vi "SMU_Meas and Calculate Resitance.vi"(7 "Current  Level":dbl=0.01, 8 "error in (no error)":errorcluster, 9 "Published Data Id":string, 10 "Pins":string[](array[string]), 11 "Semiconductor Module Context":T1) -> (0 "error Out":errorcluster, 2 "R Array":dbl[](array[numeric]), 3 "Semiconductor Module Context Out":T1)   [LabVIEW 2013]
uses:
  <vilib>/NI_TestStand_SemiconductorModule/NI_TestStand_Semiconductor_Module.lvlibp/PinMap/General/SemiconductorModuleContext.ctl
  <vilib>/NI_TestStand_SemiconductorModule/NI_TestStand_Semiconductor_Module.lvlibp/PinMap/DC Power/PinsToNIDCPowerSessions.vi
  <vilib>/NI_TestStand_SemiconductorModule/NI_TestStand_Semiconductor_Module.lvlibp/PinMap/General/Publish/PublishDataDoubleFunctionalTest.vi
  <vilib>/NI_TestStand_SemiconductorModule/NI_TestStand_Semiconductor_Module.lvlibp
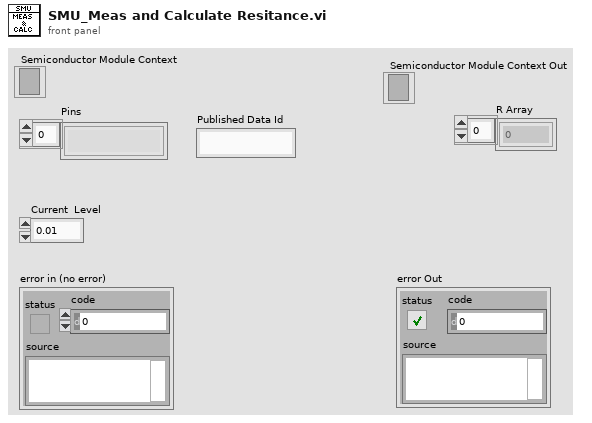
[diagram p1: front panel]
types:
  T1 = typedef "NI_TestStand_Semiconductor_Module.lvlibp/SemiconductorModuleContext.ctl" = refnum<k7>
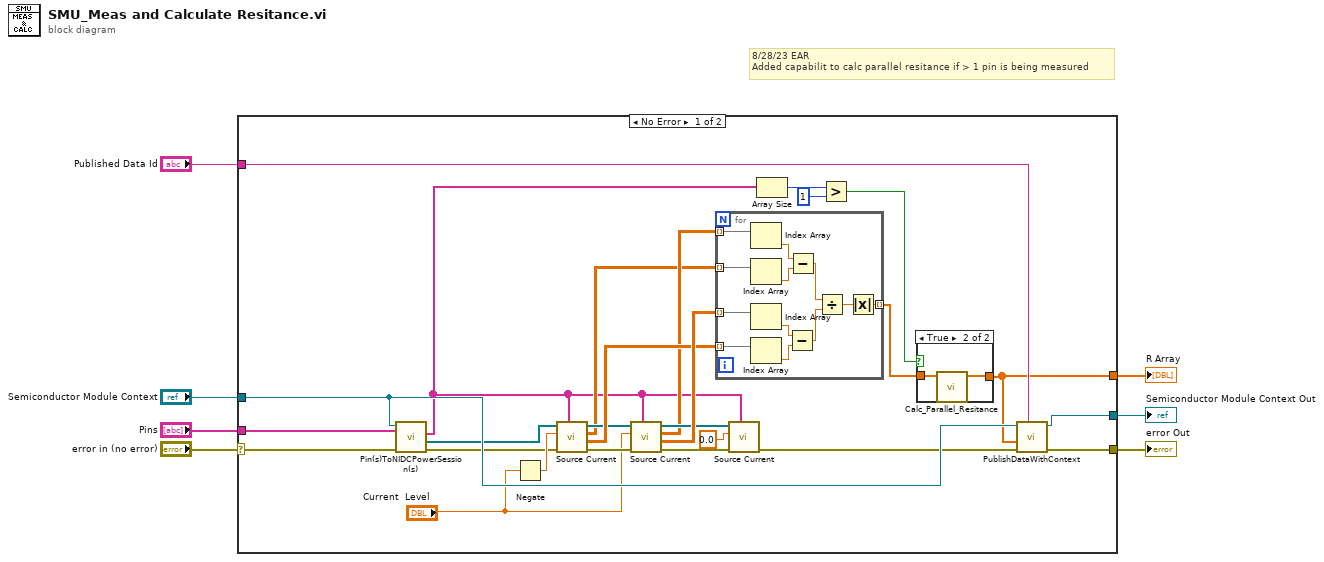
[diagram p0: block diagram]
diagram:
  # "8/28/23 EAR\nAdded capabilit to calc parallel resitance if > 1 pin is being measured"
  n1 = case shown="No Error" "error in (no error)" {
    selector: "error in (no error)" -> [w32 w50]
    tunnel: "Semiconductor Module Context" -> [w21 w49]
    tunnel: "Pins" -> [w22 _]
    tunnel: [w19 w50] -> w4
    tunnel: "Published Data Id" -> [w33 _]
    tunnel: [w27 w49] -> w2
    tunnel: [w14 _] -> w1
    frame No Error {
      n2 = call-poly <vilib>:"Pin(s)ToNIDCPowerSession(s).vi"("error in (no error)"=w32, "Pins"=w22, "Semiconductor Module Context"=w21) -> ("error out"=w10:errorcluster, "Instrument Sessions"=w9:refnum<k15>[], "Channel Lists"=w12:string[])  [unwired: 4 in, 2 out]
      n3 = Negate(x="Current  Level") -> (-x=w28:dbl)
      n4 = call "Source Current.vi"("Channel Lists"=w12, "error in (no error)"=w10, "current level"=w28, "Instrument Sessions In"=w9) -> ("error out"=w25:errorcluster, "current measurements"=w30:dbl[][], "voltage measurements"=w23:dbl[][], "Instrument Sessions Out"=w24:refnum<k15>[])  [unwired: 4 in]
      n5 = call "Source Current.vi"("Channel Lists"=w12, "error in (no error)"=w25, "current level"="Current  Level", "Instrument Sessions In"=w24) -> ("error out"=w20:errorcluster, "current measurements"=w31:dbl[][], "voltage measurements"=w26:dbl[][], "Instrument Sessions Out"=w29:refnum<k15>[])  [unwired: 4 in]
      n6 = for {
        tunnel: w26 -> [w40] mode=indexing
        tunnel: w31 -> [w48] mode=indexing
        tunnel: [w46] -> w15 mode=indexing
        tunnel: w30 -> [w44] mode=indexing
        tunnel: w23 -> [w37] mode=indexing
        n7 = Index Array(array=w40) -> (element=w39:dbl)  [unwired: 1 in]
        n8 = Index Array(array=w37) -> (element=w38:dbl)  [unwired: 1 in]
        n9 = Index Array(array=w48) -> (element=w41:dbl)  [unwired: 1 in]
        n10 = Index Array(array=w44) -> (element=w43:dbl)  [unwired: 1 in]
        n11 = Subtract(x=w41, y=w43) -> (x-y=w42:dbl)
        n12 = Subtract(x=w39, y=w38) -> (x-y=w45:dbl)
        n13 = Divide(x=w45, y=w42) -> (x/y=w47:dbl)
        n14 = Absolute Value(x=w47) -> (abs(x)=w46:dbl)
      }
      n15 = call "Source Current.vi"("Channel Lists"=w12, "error in (no error)"=w20, "current level"=0.0, "Instrument Sessions In"=w29) -> ("error out"=w11:errorcluster)  [unwired: 4 in, 3 out]
      n16 = Array Size(array=w12) -> (size(s)=w17:i32)
      n17 = Greater?(x=w17, y=1) -> (0:w13:bool)
      n18 = case shown="True" w13 {
        tunnel: w15 -> [w34 w36]
        tunnel: [w34 w35] -> w14
        frame False {
        }
        frame True {
          n19 = call "Calc_Parallel_Resitance.vi"("Resitance_Per Site"=w36) -> ("Parralel_Resistance"=w35:dbl[])  [unwired: 10 in]
        }
      }
      n20 = call-poly <vilib>:"PublishDataWithContext.vi"("Published Data Id"=w33, "error in (no error)"=w11, "Data In"=w14, "Semiconductor Module Context"=w21) -> ("error out"=w19:errorcluster, "Semiconductor Module Context Out"=w27:T1)  [unwired: 6 in]
    }
    frame Error {
    }
  }
  "error Out" <- w4
  "Semiconductor Module Context Out" <- w2
  "R Array" <- w1
